vi "update.vi"(0 "HGF_SVMonitor in":refnum<class "HGF_SVMonitor.lvclass">, 5 "error in (no error)":errorcluster) -> (14 "HGF_SVMonitor out":refnum<class "HGF_SVMonitor.lvclass">, 19 "error out":errorcluster)   [LabVIEW 2009]
doc: "This VI updates the HGF_SVMonitor.\nIt can execute following commands:\n\"stop\" -> toggle stop button from monitor\n\"register\" -> add new visitor to watchlist\n\"status\" -> return watchlist of monitor"
uses:
  HGF_SVMonitor.lvclass
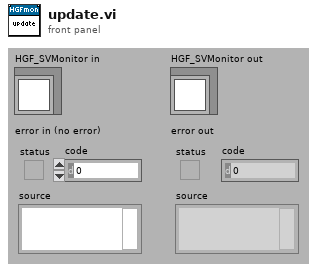
[diagram p1: front panel]
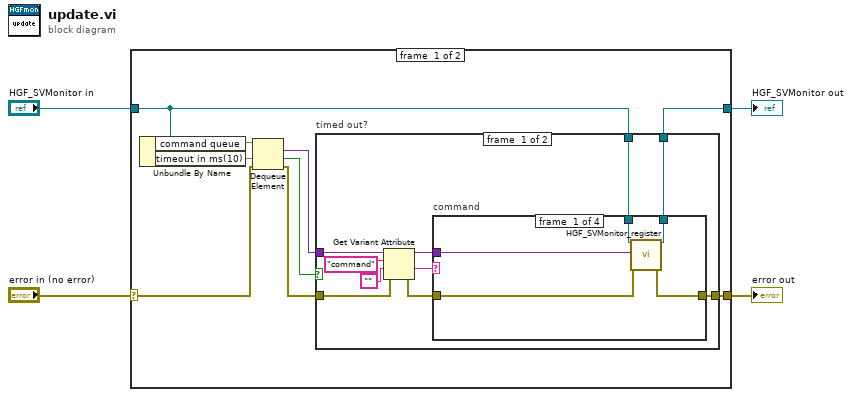
[diagram p0: block diagram]
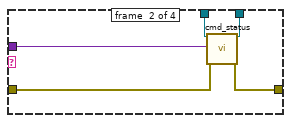
[diagram p2: hidden frame]
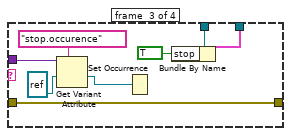
[diagram p3: hidden frame]
diagram:
  n1 = case shown="No Error" "error in (no error)" {
    selector: "error in (no error)" -> [w11 w46]
    tunnel: [w5 w47] -> w2
    tunnel: "HGF_SVMonitor in" -> [w6 w47]
    tunnel: [w7 w46] -> w1
    frame #0 {
      n2 = Unbundle By Name(w6) -> ("command queue"=w12, "timeout in ms(10)"=w13)
      n3 = Dequeue Element(queue=w12, timeout in ms (-1)=w13, error in (no error)=w11) -> (element=w9:variant, timed out?=w10:bool, error out=w8:errorcluster)  [unwired: 1 out]
      n4 = case "timed out?" shown="False" w10 {
        tunnel: w9 -> [w23 _]
        tunnel: w8 -> [w20 w45]
        tunnel: [w17 w45] -> w7
        tunnel: w6 -> [w15 w44]
        tunnel: [w14 w44] -> w5
        frame #0 {
          n5 = Get Variant Attribute(Variant=w23, name="command", default value (empty Variant)="", error in=w20) -> (duplicate Variant=w16:variant, value=w19:string, error out=w18:errorcluster)  [unwired: 1 out]
          n6 = case "command" shown="\"stop\"" w19 {
            tunnel: w18 -> [w28 w30 w38 w42]
            tunnel: [w24 w29 w38 w42] -> w17
            tunnel: w16 -> [w27 w31 w37 _]
            tunnel: w15 -> [w26 w33 w41 w43]
            tunnel: [w25 w32 w40 w43] -> w14
            frame #0 {
              n7 = call "HGF_SVMonitor_register.vi"("HGF_SVMonitor"=w26, 2:w27, "error in (no error)"=w28) -> ("HGF_SVMonitor"=w25:refnum<class "HGF_SVMonitor.lvclass">, "error out"=w24:errorcluster)  [unwired: 15 in]
            }
            frame #1 {
              n8 = call "cmd_status.vi"("HGF_SVMonitor"=w33, 2:w31, "error in (no error)"=w30) -> ("HGF_SVMonitor"=w32:refnum<class "HGF_SVMonitor.lvclass">, "error out"=w29:errorcluster)  [unwired: 15 in]
            }
            frame #2 {
              n9 = Get Variant Attribute(Variant=w37, name="stop.occurence", default value (empty Variant)=refnum<k4> refnum ("occurrence")) -> (value=w34:refnum<k4>)  [unwired: 1 in, 3 out]
              n10 = Set Occurrence(w34) -> ()
              n11 = Bundle By Name(cluster=w41, "stop"=TRUE) -> (w40:cluster{})
            }
            frame #3 {
            }
          }
        }
        frame #1 {
        }
      }
    }
    frame #1 {
    }
  }
  "error out" <- w1
  "HGF_SVMonitor out" <- w2
